vi "GenerateData.vi"(8 "error in (no error)":errorcluster, 11 "DemoCamera in":refnum<class "DemoCamera.lvclass">) -> (0 "error out":errorcluster, 2 "DataExchange":T1, 3 "DemoCamera out":refnum<class "DemoCamera.lvclass">)   [LabVIEW 2020, in "DemoCamera.lvlib" / "DemoCamera.lvclass"]
uses:
  DemoCamera.lvclass
  Hardware Abstraction Layer/Component/Device/Device/DataExchange.ctl
  Hardware Abstraction Layer/Component/Camera/Camera/Camera.lvclass
  Interface/DataListener/DataListener.lvclass
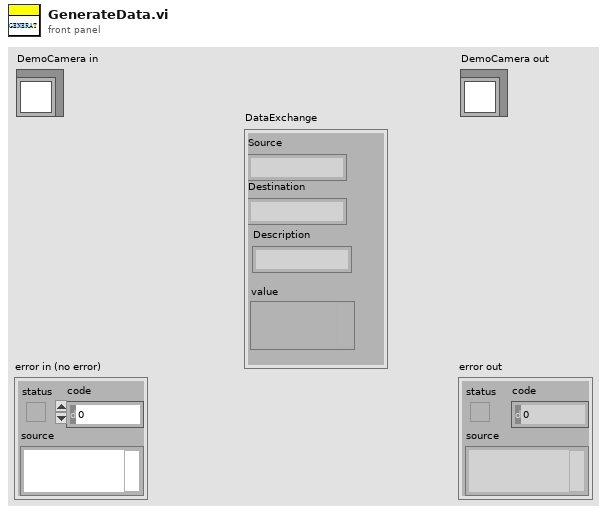
[diagram p1: front panel]
types:
  T1 = typedef "DataListener.lvclass/DataExchange.ctl" = cluster{"Source":string, "Destination":string, "Description":string, "value":variant}
  T2 = typedef "Image Type" = u32
  T3 = typedef "IMAQ Image.ctl" = refnum<image>
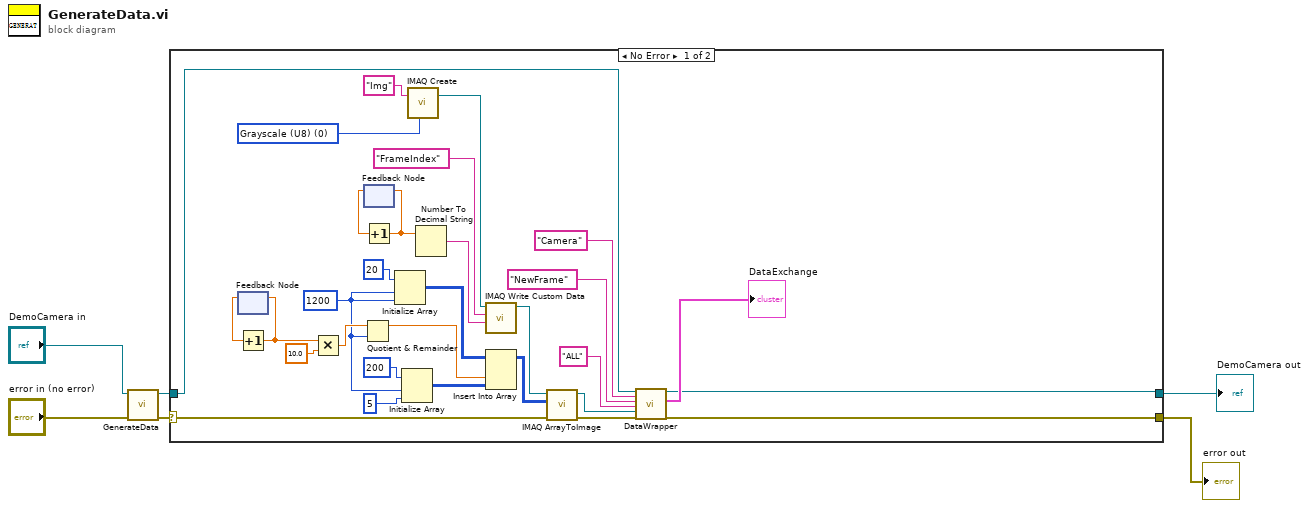
[diagram p0: block diagram]
diagram:
  n1 = call-parent "GenerateData.vi"("error in (no error)"="error in (no error)", "Device in"="DemoCamera in") -> ("error out"=w3:errorcluster, "Device out"=w4:refnum<class "DemoCamera.lvclass">)  [unwired: 7 in, 1 out]
  n2 = case shown="No Error" w3 {
    selector: w3 -> [w8 w38]
    tunnel: [w7 w38] -> w1
    tunnel: [w17 w37] -> w2
    tunnel: w4 -> [w34 w37]
    frame No Error {
      w10 = 1200 ("dimension size")
      w36 = T2 0 items=["Grayscale (U8)", "Grayscale (I16)", "Grayscale (SGL)", "Complex (CSG)", "RGB (U32)", "HSL (U32)", "RGB (U64)", "Grayscale (U16)"] ("Image Type")
      n3 = feedback #1() -> (w15:dbl)  [unwired: 1 in]
      n4 = Increment(x=w15) -> (x+1=w13:dbl)
      n5 = feedback-in #1(w13) -> ()
      n6 = Multiply(x=w13, y=10.0) -> (x*y=w12:dbl)
      n7 = Quotient & Remainder(x=w12, y=w10) -> (x-y*floor(x/y)=w14:dbl)  [unwired: 1 out]
      n8 = feedback #2() -> (w19:dbl)  [unwired: 1 in]
      n9 = Increment(x=w19) -> (x+1=w18:dbl)
      n10 = feedback-in #2(w18) -> ()
      n11 = Initialize Array(u64 20 ("element"), w10, w10) -> (w32:u64[][])
      n12 = Initialize Array(u64 200 ("element"), w10, 5 ("dimension size")) -> (w29:u64[][])
      n13 = call "IMAQ Create"("Image Name"="Img", "Image Type"=w36) -> ("New Image"=w23:T3)  [unwired: 3 in, 1 out]
      n14 = Number To Decimal String(number=w18) -> (decimal integer string=w20:string)  [unwired: 1 in]
      n15 = call "IMAQ Write Custom Data"("Custom Data In"=w20, "Key"="FrameIndex", "Image"=w23) -> ("Image Out"=w22:T3)  [unwired: 7 in, 1 out]
      n16 = Insert Into Array(array=w32, index (col)=w14, new element=w29) -> (w31:u64[][])  [unwired: 1 in]
      n17 = call "IMAQ ArrayToImage"("error in (no error)"=w8, "Image Pixels (U8)"=w31, "Image"=w22) -> ("error out"=w24:errorcluster, "Image Out"=w16:T3)  [unwired: 7 in]
      n18 = call-dynamic "DataWrapper.vi"("Device in"=w34, "Source"="Camera", "Description"="NewFrame" ("Target"), "Destination"="ALL" ("Type"), "value"=w16, "error in (no error)"=w24) -> ("Device out"=w17:refnum<class "DemoCamera.lvclass">, "DataExchange"=→"DataExchange":T1, "error out"=w7:errorcluster)  [unwired: 11 in]
    }
    frame Error {
    }
  }
  "error out" <- w1
  "DemoCamera out" <- w2
